vi "Test Child Method.vi"(8 "error in (no error)":errorcluster, 11 "Test Case Test Double Child in":refnum<class "Test Case Test Double Child.lvclass">) -> (0 "error out":errorcluster, 3 "Test Case Test Double Child out":refnum<class "Test Case Test Double Child.lvclass">)   [LabVIEW 2020, in "Test Case Test Double Child.lvclass"]
uses:
  Test Case Test Double Child.lvclass
  Test Case Test Double Child.lvclass/Test Case Test Double Child.ctl
  source/API/LUnit Test Case/LUnit Test Case.lvclass
  C:/git/astemes-lunit/tests/Test Doubles/Test Case Test Double Parent/Test Case Test Double Parent.lvclass
  C:/git/astemes-lunit/source/API/LUnit Inheriting Test Case/LUnit Test Case/LUnit Inheriting Test Case.lvclass
  C:/git/astemes-lunit/source/API/LUnit Test Case/LUnit Test Case.lvclass
  C:/git/astemes-lunit/source/Core/Runnable/Runnable.lvclass
  C:/git/astemes-lunit/tests/Test Doubles/Test Case Test Double/Test Case Test Double Child.lvclass
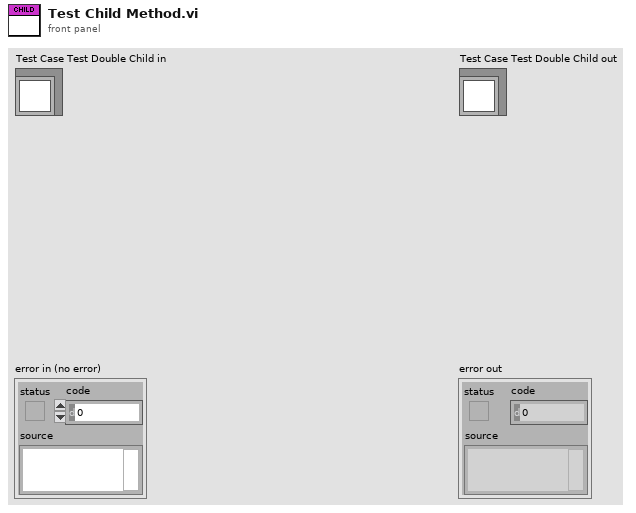
[diagram p1: front panel]
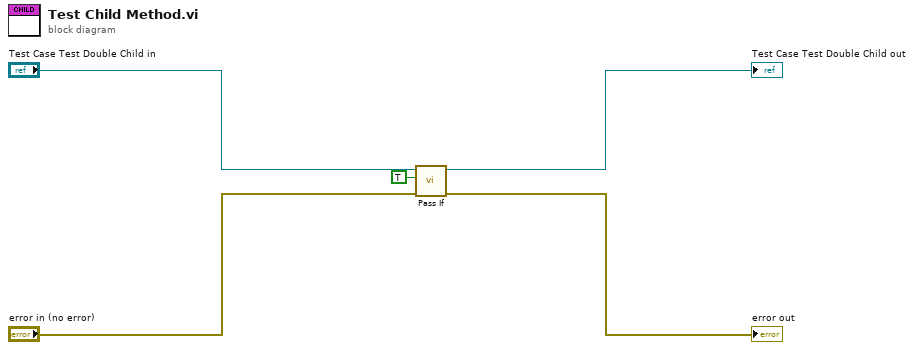
[diagram p0: block diagram]
diagram:
  n1 = call "Pass If.vi"("error in (no error)"="error in (no error)", "Pass?"=TRUE, "LUnit Test Case In"="Test Case Test Double Child in") -> ("error out"=→"error out":errorcluster, "LUnit Test Case Out"=→"Test Case Test Double Child out":refnum<class "Test Case Test Double Child.lvclass">)  [unwired: 7 in]
